vi "Newmark-QueryPosition.vi"(0 "Table VRN IN":refnum<visa-resource-name>, 7 "Bool Refnum":refnum<vi>, 11 "Error IN":errorcluster) -> (2 "X Axis":dbl, 3 "Y Axis":dbl, 4 "Table VRN OUT":refnum<visa-resource-name>, 6 "Error?":bool, 10 "Exception":string, 13 "T Axis":dbl, 14 "Z Axis":dbl, 15 "Error OUT":errorcluster)   [LabVIEW 2011]
uses:
  Comm/SerialCommError.vi
panel:
  out "ExecTime":u32
  out "N_Found":i32
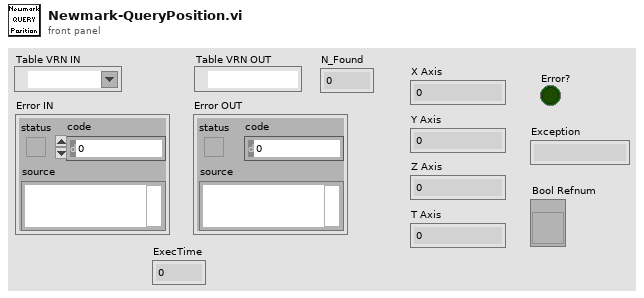
[diagram p1: front panel]
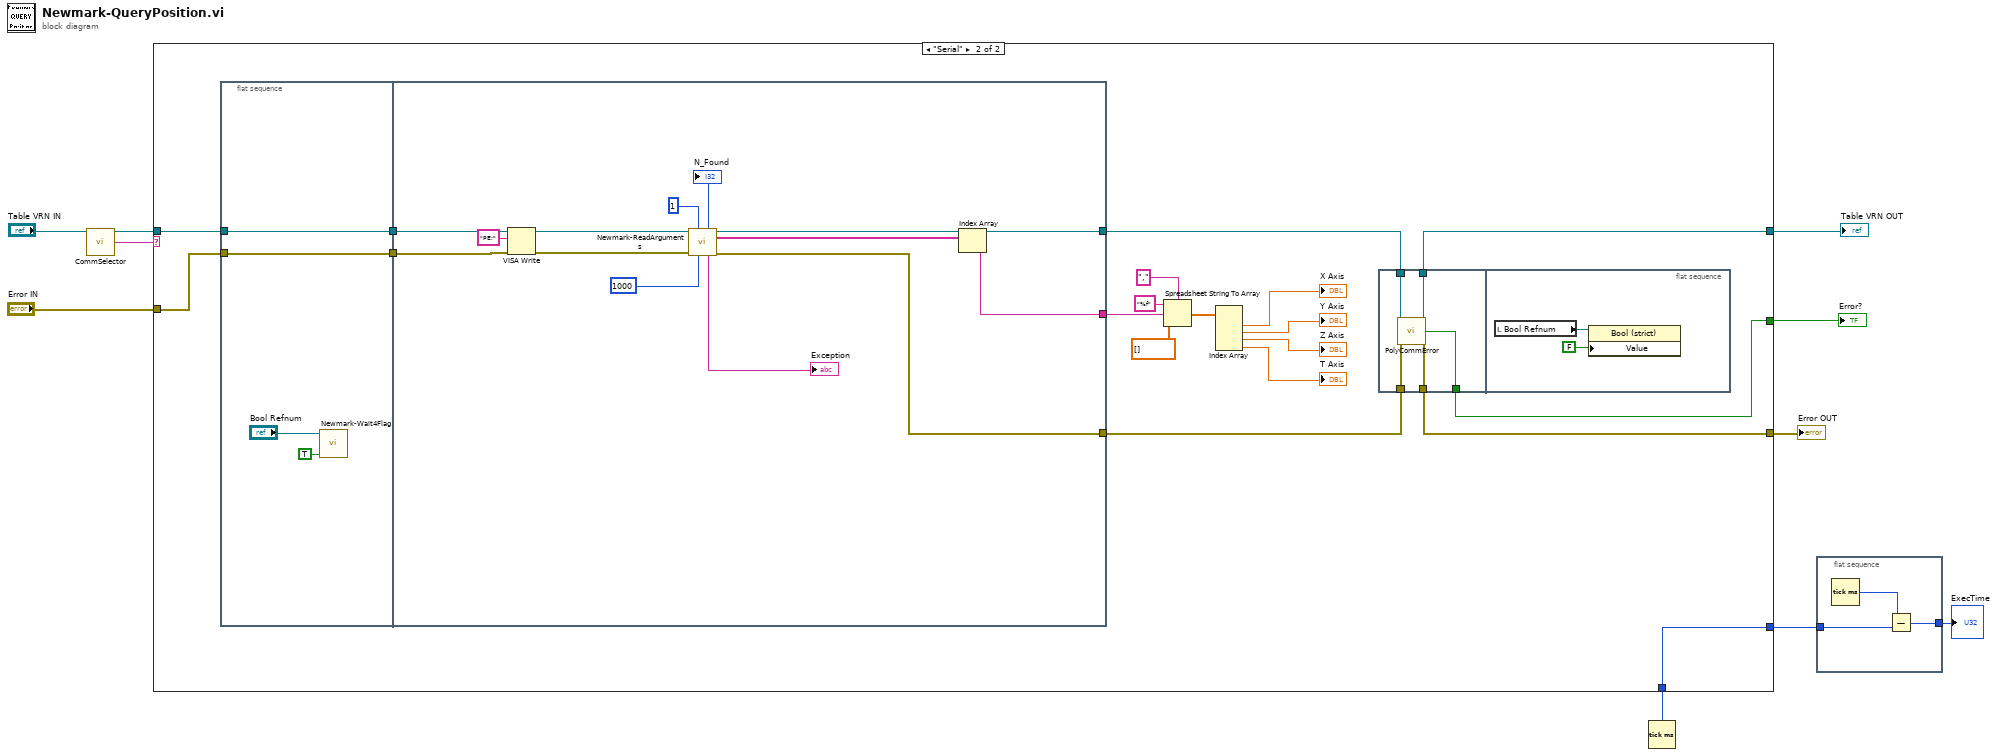
[diagram p0: block diagram]
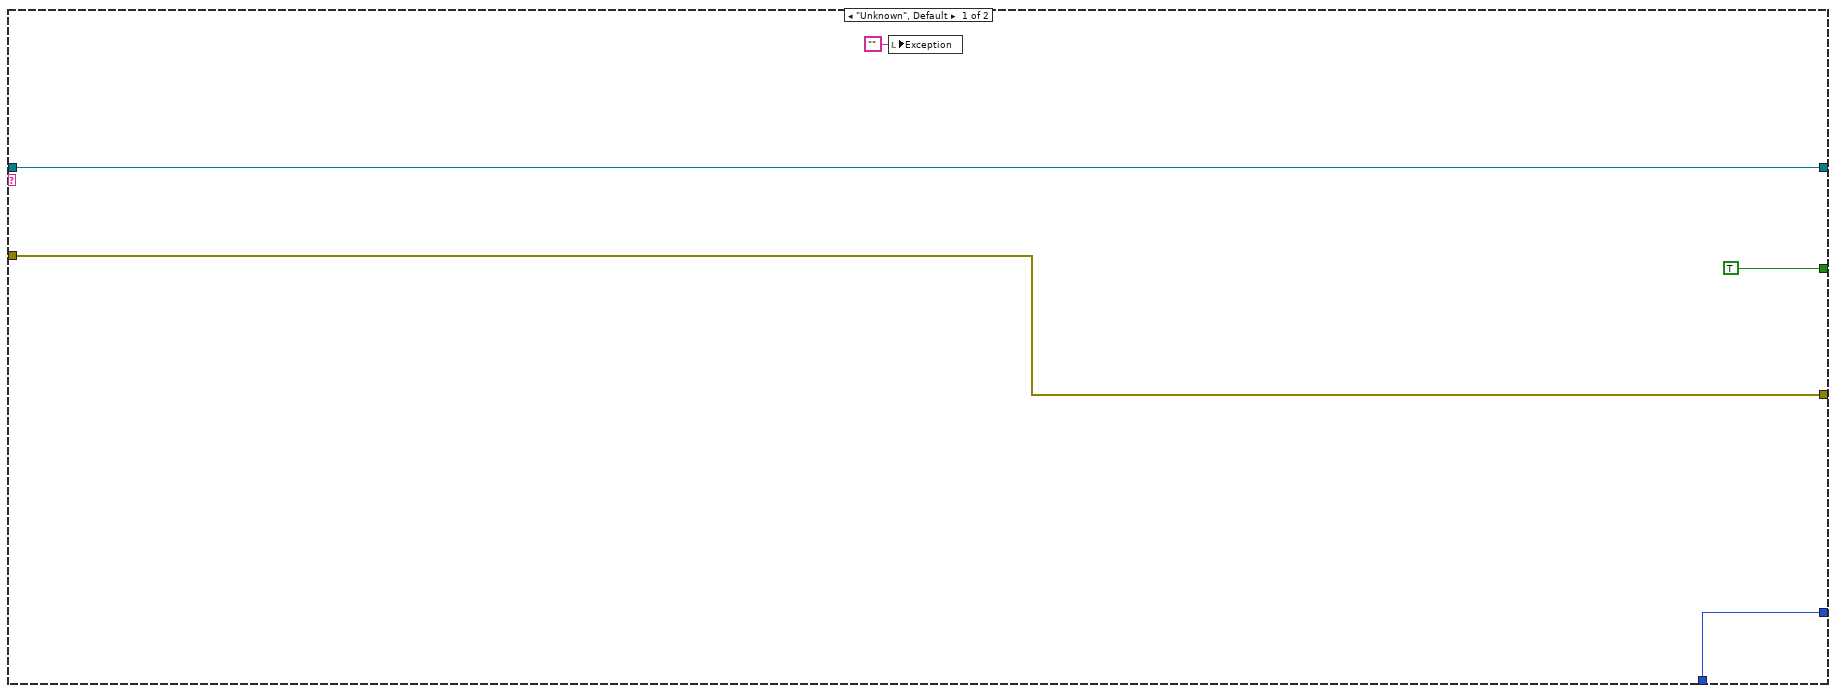
[diagram p2: hidden frame]
diagram:
  n1 = call "CommSelector.vi"("VISA resource name"="Table VRN IN") -> ("VISA resource name"=w10:refnum<visa-resource-name>, "CommType"=w5:string)  [unwired: 13 in]
  n2 = Tick Count (ms)() -> (millisecond timer value=w3:u32)
  n3 = case shown="\"Serial\"" w5 {
    tunnel: w10 -> [w15 w23]
    tunnel: "Error IN" -> [w14 w22]
    tunnel: [w14 w19] -> w7
    tunnel: [w15 w18] -> w6
    tunnel: [TRUE ("Error") w17] -> w4
    tunnel: w3 -> [w11 w16]
    tunnel: [w11 w16] -> w2
    frame "Unknown", Default {
      n4 = local write "Exception"("" ("Exception")) -> ()
    }
    frame "Serial" {
      n5 = flat-sequence {
        tunnel: w22 -> [w37]
        tunnel: w23 -> [w38]
        tunnel: [w38] -> w34
        tunnel: [w37] -> w33
        tunnel: w34 -> [w50]
        tunnel: w33 -> [w49]
        tunnel: [w51] -> w32
        tunnel: [w48] -> w21
        tunnel: [w47] -> w20
        frame #0 {
          n6 = call "Newmark-Wait4Flag.vi"("Raise Flag ?"=TRUE, "Ctl Refnum IN"="Bool Refnum") -> ()  [unwired: 8 in, 2 out]
        }
        frame #1 {
          n7 = VISA Write(VISA resource name=w50, write buffer="PE;", error in (no error)=w49) -> (VISA resource name out=w41:refnum<visa-resource-name>, error out=w40:errorcluster)  [unwired: 1 out]
          n8 = call "Newmark-ReadArguments.vi"("Table VRN IN"=w41, "N_Args"=1, "Error IN"=w40, "Timeout (ms)"=u32 1000) -> ("N_Found"=→"N_Found":i32, "Table VRN OUT"=w48:refnum<visa-resource-name>, "Args"=w44:string[], "Exception"=→"Exception":string, "Error OUT"=w47:errorcluster)  [unwired: 6 in, 1 out]
          n9 = Index Array(array=w44) -> (element=w51:string)  [unwired: 1 in]
        }
      }
      n10 = Spreadsheet String To Array(delimiter (Tab)=",", format string="%f", spreadsheet string=w32, array type (2D Dbl)=dbl[] []) -> (array=w28:dbl[])
      n11 = Index Array(array=w28) -> (element #1=→"X Axis":dbl, element #2=→"Y Axis":dbl, element #3=→"Z Axis":dbl, element #4=→"T Axis":dbl)  [unwired: 4 in]
      n12 = flat-sequence {
        tunnel: w21 -> [w55]
        tunnel: w20 -> [w56]
        tunnel: [w54] -> w18
        tunnel: [w53] -> w19
        tunnel: [w52] -> w17
        frame #0 {
          n13 = call-poly "PolyCommError.vi"("VISA IN"=w55, "error IN"=w56) -> ("VISA OUT"=w54:refnum<visa-resource-name>, "Error"=w52:bool, "error OUT"=w53:errorcluster)  [unwired: 11 in]
        }
        frame #1 {
          n14 = local read "Bool Refnum"() -> (w57:refnum<vi>)
          n15 = property on="Property Node" class="Bool (strict)"(reference=w57, "Value"=FALSE) -> ()  [unwired: 1 in, 2 out]
        }
      }
    }
  }
  "Table VRN OUT" <- w6
  "Error OUT" <- w7
  "Error?" <- w4
  n16 = flat-sequence {
    tunnel: w2 -> [w60]
    tunnel: [w59] -> w1
    frame #0 {
      n17 = Tick Count (ms)() -> (millisecond timer value=w61:u32)
      n18 = Subtract(x=w61, y=w60) -> (x-y=w59:u32)
    }
  }
  "ExecTime" <- w1
